vi "Get Mainframe VISA.vi"(8 "Error In":errorcluster, 10 "Crate":i32, 11 "VISA In":refnum<visa-resource-name>) -> (0 "Error Out":errorcluster, 2 "Version Output":string, 3 "VISA out":refnum<visa-resource-name>)   [LabVIEW 2018]
doc: "If either Mainframe VISA global variable is valid, this VI will return the requested global variable (even if that VISA is invalid). \nOnly if NEITHER global variable is valid will it use the VISA In terminal and issue the 'M' command to select the mainframe from a daisy chained set."
uses:
  archive/CAEN_SY527 v3/CAEN_SY527/CAEN globals.vi
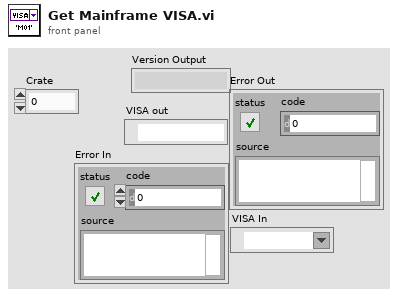
[diagram p1: front panel]
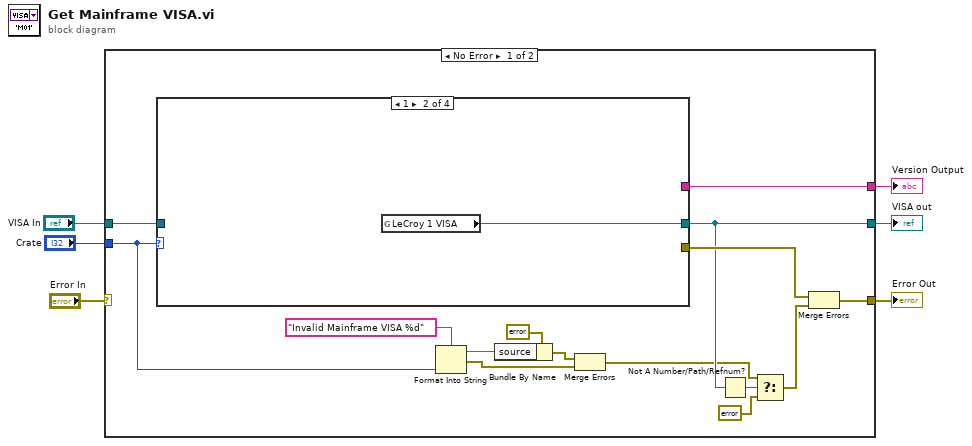
[diagram p0: block diagram]
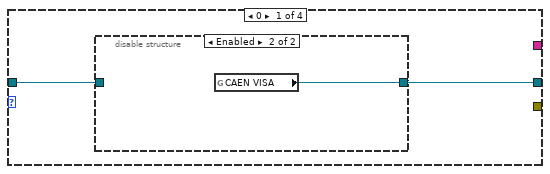
[diagram p2: hidden frame]
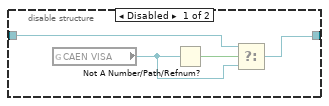
[diagram p3: hidden frame]
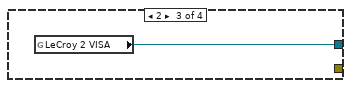
[diagram p4: hidden frame]
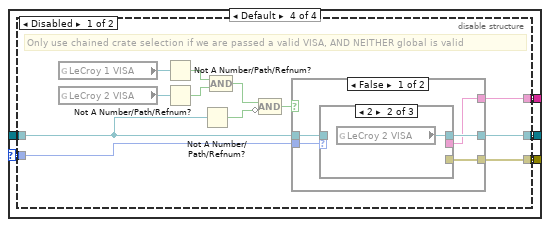
[diagram p5: hidden frame]
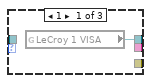
[diagram p6: hidden frame]
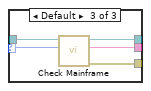
[diagram p7: hidden frame]
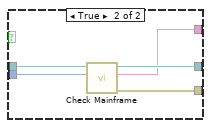
[diagram p8: hidden frame]
diagram:
  n1 = case shown="No Error" "Error In" {
    selector: "Error In" -> [_ w66]
    tunnel: "Crate" -> [w7 _]
    tunnel: [w18 w66] -> w6
    tunnel: [w19 w65] -> w4
    tunnel: "VISA In" -> [w21 w65]
    tunnel: [w17 _] -> w1
    frame No Error {
      n2 = case shown="1" w7 {
        selector: w7 -> [_ _ _ w31]
        tunnel: w21 -> [w23 _ _ w35]
        tunnel: [_ _ _ w34] -> w20
        tunnel: [w22 w29 w30 w33] -> w19
        tunnel: [_ _ _ w32] -> w17
        frame 0 {
          n3 = disable-structure shown="Enabled" {
            disable-tunnel: w23 -> [w25 _]
            disable-tunnel: [w24 w28] -> w22
            frame Disabled {
              n4 = global read "CAEN globals.vi" "CAEN VISA"() -> (w26:refnum<visa-resource-name>)
              n5 = Not A Number/Path/Refnum?(number/path/refnum=w26) -> (NaN/Path/Refnum?=w27:bool)
              n6 = Select(t=w25, s=w27, f=w26) -> (s? t:f=w24:refnum<visa-resource-name>)
            }
            frame Enabled {
              n7 = global read "CAEN globals.vi" "CAEN VISA"() -> (w28:refnum<visa-resource-name>)
            }
          }
        }
        frame 1 {
          n8 = global read "CAEN globals.vi" "LeCroy 1 VISA"() -> (w29:refnum<visa-resource-name>)
        }
        frame 2 {
          n9 = global read "CAEN globals.vi" "LeCroy 2 VISA"() -> (w30:refnum<visa-resource-name>)
        }
        frame Default {
          n10 = disable-structure shown="Disabled" {
            disable-tunnel: w35 -> [w42 _]
            disable-tunnel: [w41 _] -> w34
            disable-tunnel: [w40 _] -> w33
            disable-tunnel: [w39 _] -> w32
            disable-tunnel: w31 -> [w36 _]
            frame Disabled {
              # "Only use chained crate selection if we are passed a valid VISA, AND NEITHER global is valid"
              n11 = global read "CAEN globals.vi" "LeCroy 1 VISA"() -> (w38:refnum<visa-resource-name>)
              n12 = global read "CAEN globals.vi" "LeCroy 2 VISA"() -> (w37:refnum<visa-resource-name>)
              n13 = Not A Number/Path/Refnum?(number/path/refnum=w38) -> (NaN/Path/Refnum?=w47:bool)
              n14 = Not A Number/Path/Refnum?(number/path/refnum=w37) -> (NaN/Path/Refnum?=w46:bool)
              n15 = Not A Number/Path/Refnum?(number/path/refnum=w42) -> (NaN/Path/Refnum?=w44:bool)
              n16 = Compound Arithmetic op=AND(w47, w46) -> (w45:bool)
              n17 = Compound Arithmetic op=AND(w45, invert w44) -> (w43:bool)
              n18 = case shown="False" w43 {
                tunnel: w42 -> [w50 w64]
                tunnel: w36 -> [w51 w63]
                tunnel: [w49 w62] -> w41
                tunnel: [w52 w61] -> w40
                tunnel: [w48 w60] -> w39
                frame False {
                  n19 = case shown="2" w51 {
                    selector: w51 -> [_ _ w59]
                    tunnel: [w53 w54 w57] -> w52
                    tunnel: w50 -> [_ _ w58]
                    tunnel: [_ _ w56] -> w49
                    tunnel: [_ _ w55] -> w48
                    frame 1 {
                      n20 = global read "CAEN globals.vi" "LeCroy 1 VISA"() -> (w53:refnum<visa-resource-name>)
                    }
                    frame 2 {
                      n21 = global read "CAEN globals.vi" "LeCroy 2 VISA"() -> (w54:refnum<visa-resource-name>)
                    }
                    frame Default {
                      n22 = call "Check Mainframe.vi"("Mainframe"=w59, "VISA resource name"=w58) -> ("error out"=w56:errorcluster, "Version Output"=w55:string, "VISA resource name out"=w57:refnum<visa-resource-name>)  [unwired: 7 in]
                    }
                  }
                }
                frame True {
                  n23 = call "Check Mainframe.vi"("Mainframe"=w63, "VISA resource name"=w64) -> ("error out"=w62:errorcluster, "Version Output"=w60:string, "VISA resource name out"=w61:refnum<visa-resource-name>)  [unwired: 7 in]
                }
              }
            }
            frame Enabled {
            }
          }
        }
      }
      n24 = Format Into String(format string="Invalid Mainframe VISA %d" ("source"), w7) -> (resulting string=w13:string, error out=w15:errorcluster)  [unwired: 2 in]
      n25 = Bundle By Name(cluster=errorcluster {"status"=TRUE, "code"=0, "source"=""} ("error constant"), "source"=w13) -> (w12:errorcluster)
      n26 = Merge Errors(w12, w15) -> (w8:errorcluster)
      n27 = Not A Number/Path/Refnum?(number/path/refnum=w19) -> (NaN/Path/Refnum?=w11:bool)
      n28 = Select(t=w8, s=w11, f=errorcluster {"status"=FALSE, "code"=0, "source"=""} ("error constant")) -> (s? t:f=w9:errorcluster)
      n29 = Merge Errors(w20, w9) -> (w18:errorcluster)
    }
    frame Error {
    }
  }
  "Error Out" <- w6
  "VISA out" <- w4
  "Version Output" <- w1
